vi "DatasheetPrinter.vi"(8 "Temp":i32[](array[numeric]), 9 "Retest":i32[](array[numeric]), 10 "Data_P_F":i8[](array[numeric]), 11 "Data":sgl[](array[numeric])) -> ()   [LabVIEW 2023]
uses:
  Datasheet.ctl
panel:
  in  "Log Name":string
  in  "SN":string
  in  "Tube Type":string
  in  "Operator":string
  in  "Datasheet":T1={"Large FS Tests"=0, "Small FS Tests"=1, "TYPE:"="", "SN:"="", "Retest1"="0", "C"=0.0, "Retest2"="0", "C2"=0.0, "Retest3"="0", "C3"=0.0, "Retest4"="0", "C4"=0.0, "Retest5"="0", "C5"=0.0, "Retest6"="0", "C6"=0.0, "Retest7"="0", "C7"=0.0, "Retest10"="0", "C10"=0.0, "Retest13"="0", "C13"=0.0, "Retest19"="0", "C19"=0.0, "Retest25"="0", "C25"=0.0, "Retest29"="0", "C29"=0.0, "Retest33"="0", "C33"=0.0, "Retest37"="0", "C37"=0.0, "Retest41"="0", "C41"=0.0, "Retest45"="0", "C45"=0.0, "Retest57"="0", "C57"=0.0, "Retest61"="0", "C61"=0.0, "Log Name:"="", "Date"="", "Time"="", "OP:"=""}
  # "Temp"
  # "01"
  # "02"
  # "03"
  # "04"
  # "05"
  # "06"
  # "08"
  # "09"
  # "07"
  # "11"
  # "12"
  # "10"
  # "14"
  # "15"
  # "13"
  # "20"
  # "21"
  # "19"
  # "26"
  # "27"
  # "28"
  # "25"
  # "30"
  # "31"
  # "29"
  # "32"
  # "34"
  # "35"
  # "33"
  # "36"
  # "38"
  # "39"
  # "37"
  # "40"
  # "42"
  # "43"
  # "41"
  # "44"
  # "46"
  # "47"
  # "45"
  # "48"
  # "58"
  # "59"
  # "60"
  # "57"
  # "62"
  # "63"
  # "64"
  # "61"
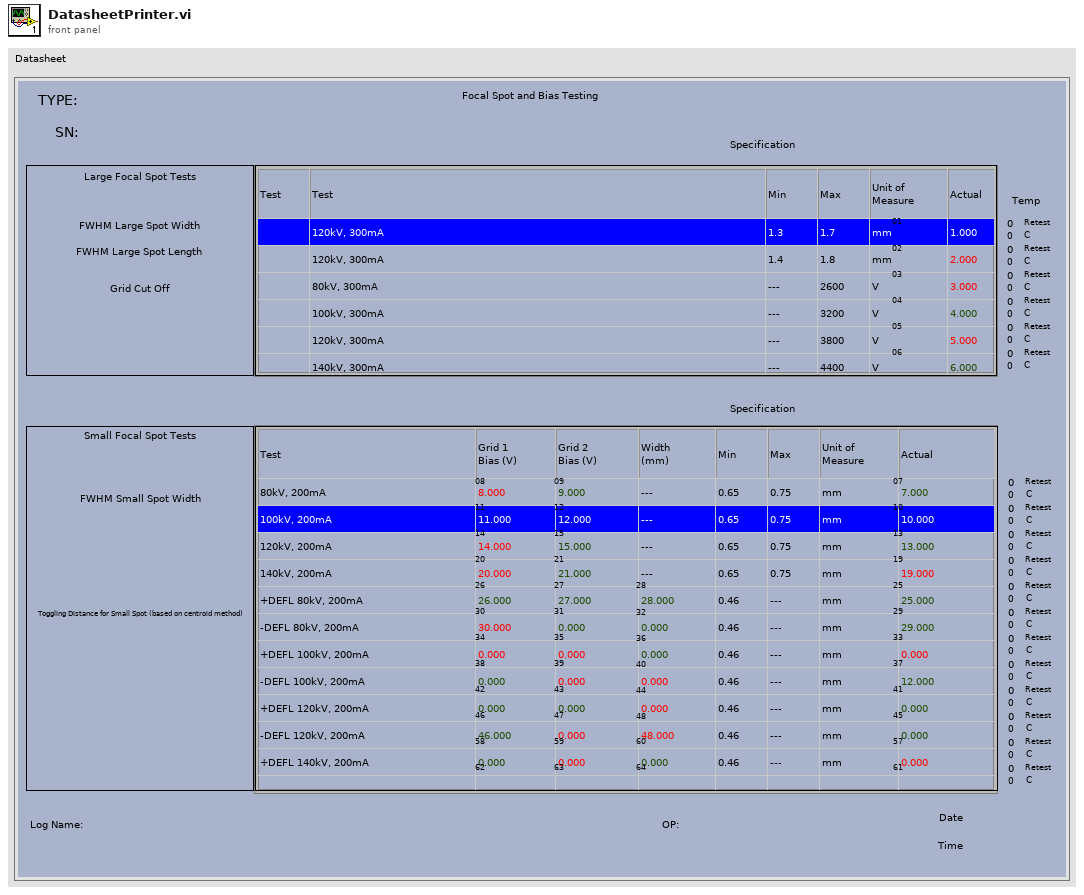
[diagram p1: front panel]
types:
  T1 = typedef "Datasheet.ctl" = cluster{"Large FS Tests":i32, "Small FS Tests":i32, "TYPE:":string, "SN:":string, "Retest1":string, "C":dbl, "Retest2":string, "C2":dbl, "Retest3":string, "C3":dbl, "Retest4":string, "C4":dbl, "Retest5":string, "C5":dbl, "Retest6":string, "C6":dbl, "Retest7":string, "C7":dbl, "Retest10":string, "C10":dbl, "Retest13":string, "C13":dbl, "Retest19":string, "C19":dbl, "Retest25":string, "C25":dbl, "Retest29":string, "C29":dbl, "Retest33":string, "C33":dbl, "Retest37":string, "C37":dbl, "Retest41":string, "C41":dbl, "Retest45":string, "C45":dbl, "Retest57":string, "C57":dbl, "Retest61":string, "C61":dbl, "Log Name:":string, "Date":string, "Time":string, "OP:":string}
  T2 = cluster{"Temp[0]":i32, "Temp[1]":i32, "Temp[2]":i32, "Temp[3]":i32, "Temp[4]":i32, "Temp[5]":i32, "Temp[6]":i32, "Temp[7]":i32, "Temp[8]":i32, "Temp[9]":i32, "Temp[10]":i32, "Temp[11]":i32, "Temp[12]":i32, "Temp[13]":i32, "Temp[14]":i32, "Temp[15]":i32, "Temp[16]":i32, "Temp[17]":i32}
  T3 = cluster{"[0]":string, "[1]":string, "[2]":string, "[3]":string, "[4]":string, "[5]":string, "[6]":string, "[7]":string, "[8]":string, "[9]":string, "[10]":string, "[11]":string, "[12]":string, "[13]":string, "[14]":string, "[15]":string, "[16]":string, "[17]":string}
  T4 = typedef "LVRowAndColumnTypeDef.ctl" = cluster{"Row":i32, "Column":i32}
  T5 = typedef "imagedata.ctl" = cluster{"image type":i32, "image depth":i32, "image":u8[], "mask":u8[], "colors":u32[], "Rectangle":cluster{"left":i16, "top":i16, "right":i16, "bottom":i16}}
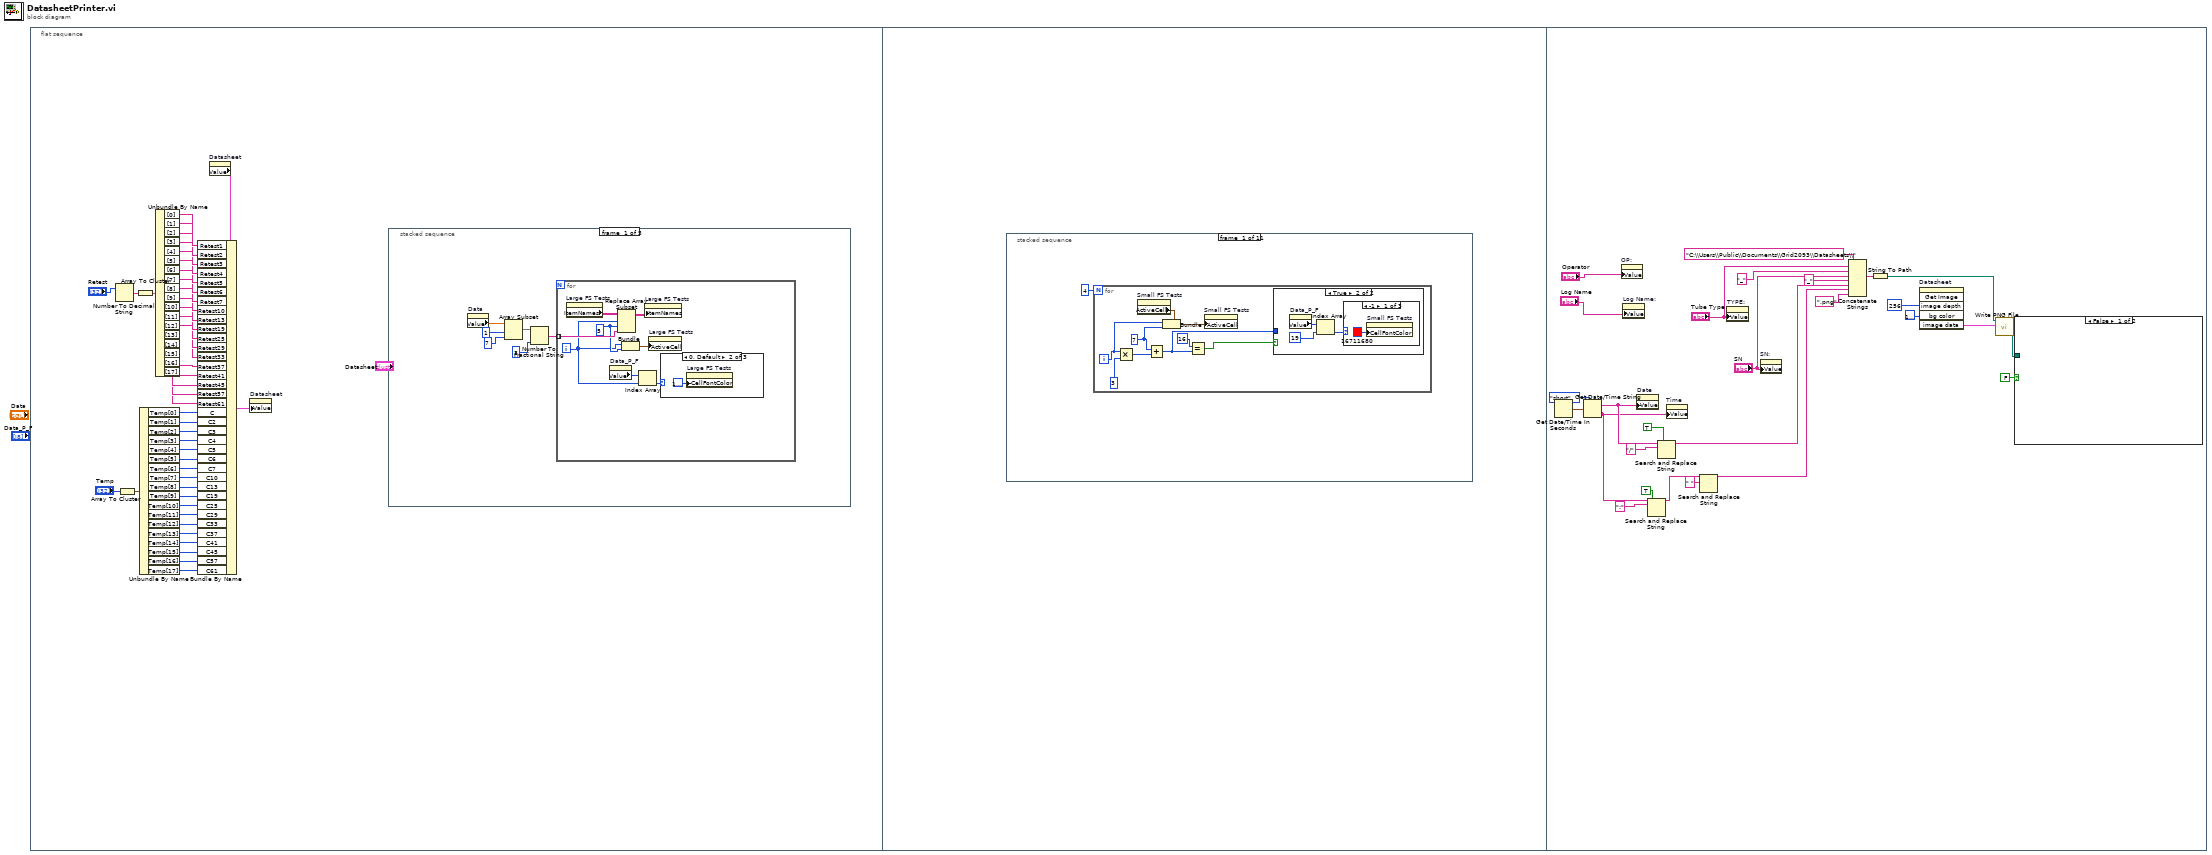
[diagram p0: block diagram]
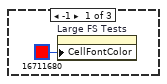
[diagram p2: hidden frame]
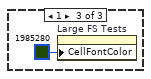
[diagram p3: hidden frame]
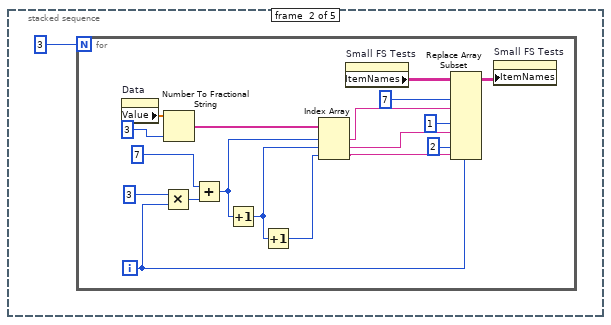
[diagram p4: hidden frame]
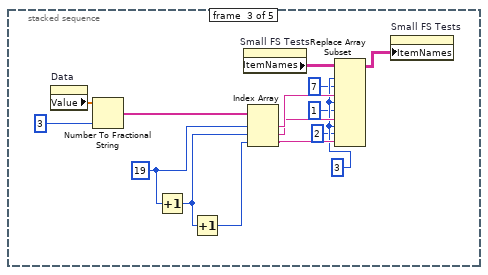
[diagram p5: hidden frame]
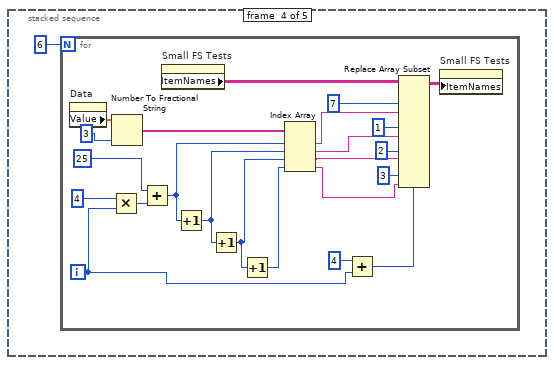
[diagram p6: hidden frame]
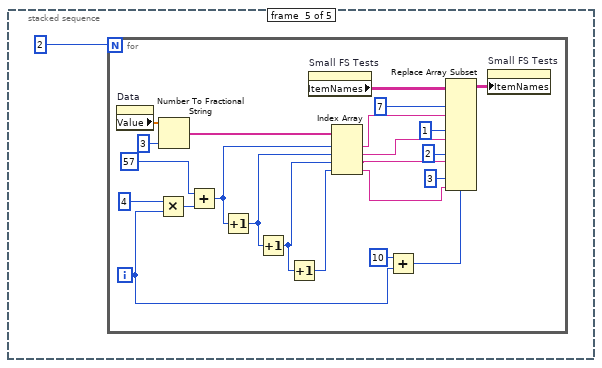
[diagram p7: hidden frame]
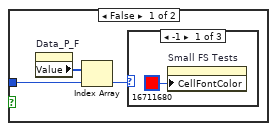
[diagram p8: hidden frame]
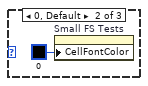
[diagram p9: hidden frame]
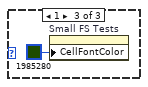
[diagram p10: hidden frame]
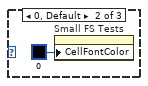
[diagram p11: hidden frame]
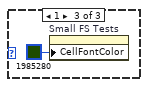
[diagram p12: hidden frame]
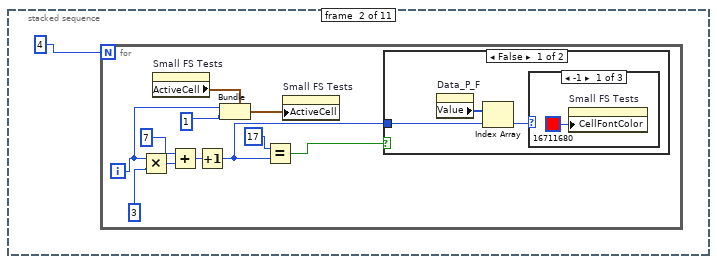
[diagram p13: hidden frame]
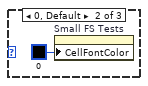
[diagram p14: hidden frame]
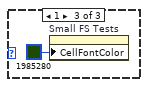
[diagram p15: hidden frame]
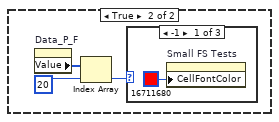
[diagram p16: hidden frame]
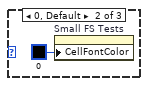
[diagram p17: hidden frame]
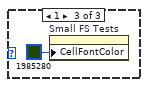
[diagram p18: hidden frame]
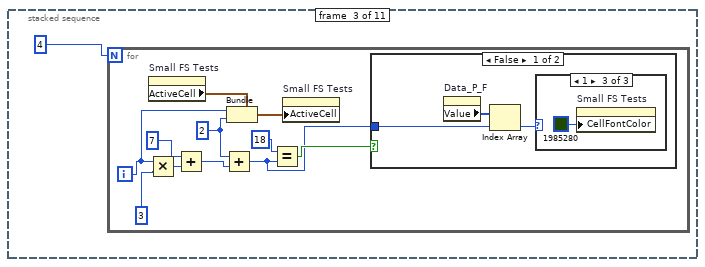
[diagram p19: hidden frame]
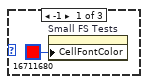
[diagram p20: hidden frame]
diagram:
  n1 = flat-sequence {
    frame #0 {
      n2 = Number To Decimal String(number="Retest") -> (decimal integer string=w40:string[])  [unwired: 1 in]
      n3 = Array To Cluster(array="Temp") -> (cluster=w19:T2)
      n4 = Array To Cluster(array=w40) -> (cluster=w39:T3)
      n5 = Unbundle By Name(w19) -> ("Temp[0]"=w18:i32, "Temp[1]"=w17:i32, "Temp[2]"=w16:i32, "Temp[3]"=w15:i32, "Temp[4]"=w14:i32, "Temp[5]"=w13:i32, "Temp[6]"=w12:i32, "Temp[7]"=w11:i32, "Temp[8]"=w10:i32, "Temp[9]"=w9:i32, "Temp[10]"=w8:i32, "Temp[11]"=w7:i32, "Temp[12]"=w6:i32, "Temp[13]"=w5:i32, "Temp[14]"=w4:i32, "Temp[15]"=w3:i32, "Temp[16]"=w2:i32, "Temp[17]"=w1:i32)
      n6 = Unbundle By Name(w39) -> ("[0]"=w38:string, "[1]"=w37:string, "[2]"=w36:string, "[3]"=w35:string, "[4]"=w34:string, "[5]"=w33:string, "[6]"=w32:string, "[7]"=w31:string, "[8]"=w30:string, "[9]"=w29:string, "[10]"=w28:string, "[11]"=w27:string, "[12]"=w26:string, "[13]"=w25:string, "[14]"=w24:string, "[15]"=w23:string, "[16]"=w22:string, "[17]"=w21:string)
      n7 = property on="Datasheet" class="Clust (strict)"() -> ("Value"=w42:T1)  [unwired: 2 in, 2 out]
      n8 = Bundle By Name(cluster=w42, "Retest1"=w38, "Retest2"=w37, "Retest3"=w36, "Retest4"=w35, "Retest5"=w34, "Retest6"=w33, "Retest7"=w32, "Retest10"=w31, "Retest13"=w30, "Retest19"=w29, "Retest25"=w28, "Retest29"=w27, "Retest33"=w26, "Retest37"=w25, "Retest41"=w24, "Retest45"=w23, "Retest57"=w22, "Retest61"=w21, "C"=w18, "C2"=w17, "C3"=w16, "C4"=w15, "C5"=w14, "C6"=w13, "C7"=w12, "C10"=w11, "C13"=w10, "C19"=w9, "C25"=w8, "C29"=w7, "C33"=w6, "C37"=w5, "C41"=w4, "C45"=w3, "C57"=w2, "C61"=w1) -> (w43:T1)
      n9 = property on="Datasheet" class="Clust (strict)"("Value"=w43) -> ()  [unwired: 2 in, 2 out]
      n10 = stacked-sequence {
        frame #0 {
          n11 = property on="Data" class="Arr (strict)"() -> ("Value"=w47:sgl[])  [unwired: 2 in, 2 out]
          n12 = Array Subset(array=w47, index=1, length=7) -> (w48:sgl[])
          n13 = Number To Fractional String(number=w48, precision (6)=i16 3) -> (F-format string=w49:string[])  [unwired: 2 in]
          n14 = for {
            tunnel: w49 -> [w57] mode=indexing
            i -> [w50]
            w52 = 5 ("index (col)")
            n15 = property on="Large FS Tests" class="MCListbox (strict)"() -> ("ItemNames"=w56:string[][])  [unwired: 2 in, 2 out]
            n16 = property on="Data_P_F" class="Arr (strict)"() -> ("Value"=w54:i8[])  [unwired: 2 in, 2 out]
            n17 = Replace Array Subset(array=w56, new element=w57, index (row)=w50, index (col)=w52) -> (w55:string[][])
            n18 = Bundle(w50, "index (col)"=w52) -> (w51:cluster{i32, "index (col)":i32})  [unwired: 1 in]
            n19 = Index Array(array=w54, index=w50) -> (element=w53:i8)
            n20 = property on="Large FS Tests" class="MCListbox (strict)"("ItemNames"=w55) -> ()  [unwired: 2 in, 2 out]
            n21 = property on="Large FS Tests" class="MCListbox (strict)"("ActiveCell"=w51) -> ()  [unwired: 2 in, 2 out]
            n22 = case shown="0, Default" w53 {
              frame -1 {
                n23 = property on="Large FS Tests" class="MCListbox (strict)"("CellFontColor"=u32 16711680 ("Active Cell:Cell Font:Color")) -> ()  [unwired: 2 in, 2 out]
              }
              frame 0, Default {
                n24 = property on="Large FS Tests" class="MCListbox (strict)"("CellFontColor"=u32 16777222 ("Active Cell:Cell Font:Color")) -> ()  [unwired: 2 in, 2 out]
              }
              frame 1 {
                n25 = property on="Large FS Tests" class="MCListbox (strict)"("CellFontColor"=u32 1985280 ("Active Cell:Cell Font:Color")) -> ()  [unwired: 2 in, 2 out]
              }
            }
          }
        }
        frame #1 {
          n26 = for {
            N: 3 -> [_]
            i -> [w68]
            n27 = property on="Data" class="Arr (strict)"() -> ("Value"=w74:sgl[])  [unwired: 2 in, 2 out]
            n28 = Multiply(x=3, y=w68) -> (x*y=w76:i32)
            n29 = Number To Fractional String(number=w74, precision (6)=i16 3) -> (F-format string=w73:string[])  [unwired: 2 in]
            n30 = Add(x=7, y=w76) -> (x+y=w75:i32)
            n31 = Increment(x=w75) -> (x+1=w67:i32)
            n32 = Increment(x=w67) -> (x+1=w66:i32)
            n33 = Index Array(array=w73, index #1=w75, index #2=w67, index #3=w66) -> (element #1=w72:string, element #2=w65:string, element #3=w64:string)
            n34 = property on="Small FS Tests" class="MCListbox (strict)"() -> ("ItemNames"=w79:string[][])  [unwired: 2 in, 2 out]
            n35 = Replace Array Subset(array=w79, new element #1=w72, index (row) #1=w68, index (col) #1=7 ("index (col)"), new element #2=w65, index (row) #2=w68, index (col) #2=1 ("index (col)"), new element #3=w64, index (row) #3=w68, index (col) #3=2 ("index (col)")) -> (w62:string[][])
            n36 = property on="Small FS Tests" class="MCListbox (strict)"("ItemNames"=w62) -> ()  [unwired: 2 in, 2 out]
          }
        }
        frame #2 {
          w84 = 19 ("x")
          w83 = 3 ("index (row)")
          n37 = property on="Data" class="Arr (strict)"() -> ("Value"=w92:sgl[])  [unwired: 2 in, 2 out]
          n38 = Number To Fractional String(number=w92, precision (6)=i16 3) -> (F-format string=w91:string[])  [unwired: 2 in]
          n39 = Increment(x=w84) -> (x+1=w89:i32)
          n40 = Increment(x=w89) -> (x+1=w88:i32)
          n41 = property on="Small FS Tests" class="MCListbox (strict)"() -> ("ItemNames"=w93:string[][])  [unwired: 2 in, 2 out]
          n42 = Index Array(array=w91, index #1=w84, index #2=w89, index #3=w88) -> (element #1=w90:string, element #2=w87:string, element #3=w86:string)
          n43 = Replace Array Subset(array=w93, new element #1=w90, index (row) #1=w83, index (col) #1=7 ("index (col)"), new element #2=w87, index (row) #2=w83, index (col) #2=1 ("index (col)"), new element #3=w86, index (row) #3=w83, index (col) #3=2 ("index (col)")) -> (w94:string[][])
          n44 = property on="Small FS Tests" class="MCListbox (strict)"("ItemNames"=w94) -> ()  [unwired: 2 in, 2 out]
        }
        frame #3 {
          n45 = for {
            N: 6 -> [_]
            i -> [w100]
            n46 = property on="Data" class="Arr (strict)"() -> ("Value"=w114:sgl[])  [unwired: 2 in, 2 out]
            n47 = Multiply(x=4, y=w100) -> (x*y=w116:i32)
            n48 = Number To Fractional String(number=w114, precision (6)=i16 3) -> (F-format string=w113:string[])  [unwired: 2 in]
            n49 = Add(x=25, y=w116) -> (x+y=w115:i32)
            n50 = property on="Small FS Tests" class="MCListbox (strict)"() -> ("ItemNames"=w96:string[][])  [unwired: 2 in, 2 out]
            n51 = Increment(x=w115) -> (x+1=w108:i32)
            n52 = Increment(x=w108) -> (x+1=w104:i32)
            n53 = Increment(x=w104) -> (x+1=w103:i32)
            n54 = Index Array(array=w113, index #1=w115, index #2=w108, index #3=w104, index #4=w103) -> (element #1=w112:string, element #2=w107:string, element #3=w106:string, element #4=w102:string)
            n55 = Add(x=4, y=w100) -> (x+y=w99:i32)
            n56 = Replace Array Subset(array=w96, new element #1=w112, index (row) #1=w99, index (col) #1=7 ("index (col)"), new element #2=w107, index (row) #2=w99, index (col) #2=1 ("index (col)"), new element #3=w106, index (row) #3=w99, index (col) #3=2 ("index (col)"), new element #4=w102, index (row) #4=w99, index (col) #4=3 ("index (col)")) -> (w97:string[][])
            n57 = property on="Small FS Tests" class="MCListbox (strict)"("ItemNames"=w97) -> ()  [unwired: 2 in, 2 out]
          }
        }
        frame #4 {
          n58 = for {
            N: 2 -> [_]
            i -> [w123]
            n59 = property on="Data" class="Arr (strict)"() -> ("Value"=w138:sgl[])  [unwired: 2 in, 2 out]
            n60 = Multiply(x=4, y=w123) -> (x*y=w140:i32)
            n61 = Number To Fractional String(number=w138, precision (6)=i16 3) -> (F-format string=w137:string[])  [unwired: 2 in]
            n62 = Add(x=57, y=w140) -> (x+y=w139:i32)
            n63 = Increment(x=w139) -> (x+1=w131:i32)
            n64 = Increment(x=w131) -> (x+1=w127:i32)
            n65 = Increment(x=w127) -> (x+1=w126:i32)
            n66 = property on="Small FS Tests" class="MCListbox (strict)"() -> ("ItemNames"=w120:string[][])  [unwired: 2 in, 2 out]
            n67 = Index Array(array=w137, index #1=w139, index #2=w131, index #3=w127, index #4=w126) -> (element #1=w136:string, element #2=w130:string, element #3=w129:string, element #4=w125:string)
            n68 = Add(x=10, y=w123) -> (x+y=w122:i32)
            n69 = Replace Array Subset(array=w120, new element #1=w136, index (row) #1=w122, index (col) #1=7 ("index (col)"), new element #2=w130, index (row) #2=w122, index (col) #2=1 ("index (col)"), new element #3=w129, index (row) #3=w122, index (col) #3=2 ("index (col)"), new element #4=w125, index (row) #4=w122, index (col) #4=3 ("index (col)")) -> (w132:string[][])
            n70 = property on="Small FS Tests" class="MCListbox (strict)"("ItemNames"=w132) -> ()  [unwired: 2 in, 2 out]
          }
        }
      }
    }
    frame #1 {
      n71 = stacked-sequence {
        frame #0 {
          n72 = for {
            N: 4 -> [_]
            i -> [w145]
            w148 = 7 ("x")
            n73 = Multiply(x=w145, y=3 ("x")) -> (x*y=w152:i32)
            n74 = property on="Small FS Tests" class="MCListbox (strict)"() -> ("ActiveCell"=w144:T4)  [unwired: 2 in, 2 out]
            n75 = Add(x=w148, y=w152) -> (x+y=w146:i32)
            n76 = Bundle(cluster=w144, "Row"=w145, "Column"=w148) -> (w147:T4)
            n77 = Equal?(x=16, y=w146) -> (x = y?=w150:bool)
            n78 = property on="Small FS Tests" class="MCListbox (strict)"("ActiveCell"=w147) -> ()  [unwired: 2 in, 2 out]
            n79 = case shown="True" w150 {
              tunnel: w146 -> [w154 _]
              frame False {
                n80 = property on="Data_P_F" class="Arr (strict)"() -> ("Value"=w155:i8[])  [unwired: 2 in, 2 out]
                n81 = Index Array(array=w155, index=w154) -> (element=w153:i8)
                n82 = case shown="-1" w153 {
                  frame -1 {
                    n83 = property on="Small FS Tests" class="MCListbox (strict)"("CellFontColor"=u32 16711680 ("Active Cell:Cell Font:Color")) -> ()  [unwired: 2 in, 2 out]
                  }
                  frame 0, Default {
                    n84 = property on="Small FS Tests" class="MCListbox (strict)"("CellFontColor"=u32 0 ("Active Cell:Cell Font:Color")) -> ()  [unwired: 2 in, 2 out]
                  }
                  frame 1 {
                    n85 = property on="Small FS Tests" class="MCListbox (strict)"("CellFontColor"=u32 1985280 ("Active Cell:Cell Font:Color")) -> ()  [unwired: 2 in, 2 out]
                  }
                }
              }
              frame True {
                n86 = property on="Data_P_F" class="Arr (strict)"() -> ("Value"=w161:i8[])  [unwired: 2 in, 2 out]
                n87 = Index Array(array=w161, index=19) -> (element=w160:i8)
                n88 = case shown="-1" w160 {
                  frame -1 {
                    n89 = property on="Small FS Tests" class="MCListbox (strict)"("CellFontColor"=u32 16711680 ("Active Cell:Cell Font:Color")) -> ()  [unwired: 2 in, 2 out]
                  }
                  frame 0, Default {
                    n90 = property on="Small FS Tests" class="MCListbox (strict)"("CellFontColor"=u32 0 ("Active Cell:Cell Font:Color")) -> ()  [unwired: 2 in, 2 out]
                  }
                  frame 1 {
                    n91 = property on="Small FS Tests" class="MCListbox (strict)"("CellFontColor"=u32 1985280 ("Active Cell:Cell Font:Color")) -> ()  [unwired: 2 in, 2 out]
                  }
                }
              }
            }
          }
        }
        frame #1 {
          n92 = for {
            N: 4 -> [_]
            i -> [w167]
            n93 = Multiply(x=w167, y=3 ("x")) -> (x*y=w176:i32)
            n94 = property on="Small FS Tests" class="MCListbox (strict)"() -> ("ActiveCell"=w166:T4)  [unwired: 2 in, 2 out]
            n95 = Add(x=7, y=w176) -> (x+y=w170:i32)
            n96 = Increment(x=w170) -> (x+1=w169:i32)
            n97 = Bundle(cluster=w166, "Row"=w167, "Column"=1 ("x")) -> (w171:T4)
            n98 = Equal?(x=17, y=w169) -> (x = y?=w174:bool)
            n99 = property on="Small FS Tests" class="MCListbox (strict)"("ActiveCell"=w171) -> ()  [unwired: 2 in, 2 out]
            n100 = case shown="False" w174 {
              tunnel: w169 -> [w178 _]
              frame False {
                n101 = property on="Data_P_F" class="Arr (strict)"() -> ("Value"=w179:i8[])  [unwired: 2 in, 2 out]
                n102 = Index Array(array=w179, index=w178) -> (element=w177:i8)
                n103 = case shown="-1" w177 {
                  frame -1 {
                    n104 = property on="Small FS Tests" class="MCListbox (strict)"("CellFontColor"=u32 16711680 ("Active Cell:Cell Font:Color")) -> ()  [unwired: 2 in, 2 out]
                  }
                  frame 0, Default {
                    n105 = property on="Small FS Tests" class="MCListbox (strict)"("CellFontColor"=u32 0 ("Active Cell:Cell Font:Color")) -> ()  [unwired: 2 in, 2 out]
                  }
                  frame 1 {
                    n106 = property on="Small FS Tests" class="MCListbox (strict)"("CellFontColor"=u32 1985280 ("Active Cell:Cell Font:Color")) -> ()  [unwired: 2 in, 2 out]
                  }
                }
              }
              frame True {
                n107 = property on="Data_P_F" class="Arr (strict)"() -> ("Value"=w185:i8[])  [unwired: 2 in, 2 out]
                n108 = Index Array(array=w185, index=20) -> (element=w184:i8)
                n109 = case shown="-1" w184 {
                  frame -1 {
                    n110 = property on="Small FS Tests" class="MCListbox (strict)"("CellFontColor"=u32 16711680 ("Active Cell:Cell Font:Color")) -> ()  [unwired: 2 in, 2 out]
                  }
                  frame 0, Default {
                    n111 = property on="Small FS Tests" class="MCListbox (strict)"("CellFontColor"=u32 0 ("Active Cell:Cell Font:Color")) -> ()  [unwired: 2 in, 2 out]
                  }
                  frame 1 {
                    n112 = property on="Small FS Tests" class="MCListbox (strict)"("CellFontColor"=u32 1985280 ("Active Cell:Cell Font:Color")) -> ()  [unwired: 2 in, 2 out]
                  }
                }
              }
            }
          }
        }
        frame #2 {
          n113 = for {
            N: 4 -> [_]
            i -> [w191]
            w192 = 2 ("x")
            n114 = Multiply(x=w191, y=3 ("x")) -> (x*y=w200:i32)
            n115 = property on="Small FS Tests" class="MCListbox (strict)"() -> ("ActiveCell"=w190:T4)  [unwired: 2 in, 2 out]
            n116 = Add(x=7, y=w200) -> (x+y=w193:i32)
            n117 = Add(x=w192, y=w193) -> (x+y=w194:i32)
            n118 = Bundle(cluster=w190, "Row"=w191, "Column"=w192) -> (w195:T4)
            n119 = Equal?(x=18, y=w194) -> (x = y?=w198:bool)
            n120 = property on="Small FS Tests" class="MCListbox (strict)"("ActiveCell"=w195) -> ()  [unwired: 2 in, 2 out]
            n121 = case shown="False" w198 {
              tunnel: w194 -> [w202 _]
              frame False {
                n122 = property on="Data_P_F" class="Arr (strict)"() -> ("Value"=w203:i8[])  [unwired: 2 in, 2 out]
                n123 = Index Array(array=w203, index=w202) -> (element=w201:i8)
                n124 = case shown="1" w201 {
                  frame -1 {
                    n125 = property on="Small FS Tests" class="MCListbox (strict)"("CellFontColor"=u32 16711680 ("Active Cell:Cell Font:Color")) -> ()  [unwired: 2 in, 2 out]
                  }
                  frame 0, Default {
                    n126 = property on="Small FS Tests" class="MCListbox (strict)"("CellFontColor"=u32 0 ("Active Cell:Cell Font:Color")) -> ()  [unwired: 2 in, 2 out]
                  }
                  frame 1 {
                    n127 = property on="Small FS Tests" class="MCListbox (strict)"("CellFontColor"=u32 1985280 ("Active Cell:Cell Font:Color")) -> ()  [unwired: 2 in, 2 out]
                  }
                }
              }
              frame True {
                n128 = property on="Data_P_F" class="Arr (strict)"() -> ("Value"=w209:i8[])  [unwired: 2 in, 2 out]
                n129 = Index Array(array=w209, index=21) -> (element=w208:i8)
                n130 = case shown="1" w208 {
                  frame -1 {
                    n131 = property on="Small FS Tests" class="MCListbox (strict)"("CellFontColor"=u32 16711680 ("Active Cell:Cell Font:Color")) -> ()  [unwired: 2 in, 2 out]
                  }
                  frame 0, Default {
                    n132 = property on="Small FS Tests" class="MCListbox (strict)"("CellFontColor"=u32 0 ("Active Cell:Cell Font:Color")) -> ()  [unwired: 2 in, 2 out]
                  }
                  frame 1 {
                    n133 = property on="Small FS Tests" class="MCListbox (strict)"("CellFontColor"=u32 1985280 ("Active Cell:Cell Font:Color")) -> ()  [unwired: 2 in, 2 out]
                  }
                }
              }
            }
          }
        }
        frame #3 {
          n134 = for {
            N: 6 -> [_]
            i -> [w216]
            n135 = Multiply(x=w216, y=4 ("x")) -> (x*y=w225:i32)
            n136 = Add(x=4, y=w216) -> (x+y=w217:i32)
            n137 = property on="Small FS Tests" class="MCListbox (strict)"() -> ("ActiveCell"=w214:T4)  [unwired: 2 in, 2 out]
            n138 = Add(x=25, y=w225) -> (x+y=w222:i32)
            n139 = Bundle(cluster=w214, "Row"=w217, "Column"=7) -> (w219:T4)
            n140 = property on="Small FS Tests" class="MCListbox (strict)"("ActiveCell"=w219) -> ()  [unwired: 2 in, 2 out]
            n141 = property on="Data_P_F" class="Arr (strict)"() -> ("Value"=w221:i8[])  [unwired: 2 in, 2 out]
            n142 = Index Array(array=w221, index=w222) -> (element=w220:i8)
            n143 = case shown="1" w220 {
              frame -1 {
                n144 = property on="Small FS Tests" class="MCListbox (strict)"("CellFontColor"=u32 16711680 ("Active Cell:Cell Font:Color")) -> ()  [unwired: 2 in, 2 out]
              }
              frame 0, Default {
                n145 = property on="Small FS Tests" class="MCListbox (strict)"("CellFontColor"=u32 0 ("Active Cell:Cell Font:Color")) -> ()  [unwired: 2 in, 2 out]
              }
              frame 1 {
                n146 = property on="Small FS Tests" class="MCListbox (strict)"("CellFontColor"=u32 1985280 ("Active Cell:Cell Font:Color")) -> ()  [unwired: 2 in, 2 out]
              }
            }
          }
        }
        frame #4 {
          n147 = for {
            N: 6 -> [_]
            i -> [w232]
            n148 = Multiply(x=w232, y=4 ("x")) -> (x*y=w242:i32)
            n149 = Add(x=4, y=w232) -> (x+y=w233:i32)
            n150 = property on="Small FS Tests" class="MCListbox (strict)"() -> ("ActiveCell"=w230:T4)  [unwired: 2 in, 2 out]
            n151 = Add(x=25, y=w242) -> (x+y=w239:i32)
            n152 = Bundle(cluster=w230, "Row"=w233, "Column"=1) -> (w236:T4)
            n153 = Increment(x=w239) -> (x+1=w234:i32)
            n154 = property on="Small FS Tests" class="MCListbox (strict)"("ActiveCell"=w236) -> ()  [unwired: 2 in, 2 out]
            n155 = property on="Data_P_F" class="Arr (strict)"() -> ("Value"=w238:i8[])  [unwired: 2 in, 2 out]
            n156 = Index Array(array=w238, index=w234) -> (element=w237:i8)
            n157 = case shown="1" w237 {
              frame -1 {
                n158 = property on="Small FS Tests" class="MCListbox (strict)"("CellFontColor"=u32 16711680 ("Active Cell:Cell Font:Color")) -> ()  [unwired: 2 in, 2 out]
              }
              frame 0, Default {
                n159 = property on="Small FS Tests" class="MCListbox (strict)"("CellFontColor"=u32 0 ("Active Cell:Cell Font:Color")) -> ()  [unwired: 2 in, 2 out]
              }
              frame 1 {
                n160 = property on="Small FS Tests" class="MCListbox (strict)"("CellFontColor"=u32 1985280 ("Active Cell:Cell Font:Color")) -> ()  [unwired: 2 in, 2 out]
              }
            }
          }
        }
        frame #5 {
          n161 = for {
            N: 6 -> [_]
            i -> [w249]
            n162 = Multiply(x=w249, y=4 ("x")) -> (x*y=w260:i32)
            n163 = Add(x=4, y=w249) -> (x+y=w250:i32)
            n164 = property on="Small FS Tests" class="MCListbox (strict)"() -> ("ActiveCell"=w247:T4)  [unwired: 2 in, 2 out]
            n165 = Add(x=25, y=w260) -> (x+y=w257:i32)
            n166 = Bundle(cluster=w247, "Row"=w250, "Column"=2) -> (w254:T4)
            n167 = property on="Small FS Tests" class="MCListbox (strict)"("ActiveCell"=w254) -> ()  [unwired: 2 in, 2 out]
            n168 = Add(x=w257, y=2) -> (x+y=w252:i32)
            n169 = property on="Data_P_F" class="Arr (strict)"() -> ("Value"=w256:i8[])  [unwired: 2 in, 2 out]
            n170 = Index Array(array=w256, index=w252) -> (element=w255:i8)
            n171 = case shown="-1" w255 {
              frame -1 {
                n172 = property on="Small FS Tests" class="MCListbox (strict)"("CellFontColor"=u32 16711680 ("Active Cell:Cell Font:Color")) -> ()  [unwired: 2 in, 2 out]
              }
              frame 0, Default {
                n173 = property on="Small FS Tests" class="MCListbox (strict)"("CellFontColor"=u32 0 ("Active Cell:Cell Font:Color")) -> ()  [unwired: 2 in, 2 out]
              }
              frame 1 {
                n174 = property on="Small FS Tests" class="MCListbox (strict)"("CellFontColor"=u32 1985280 ("Active Cell:Cell Font:Color")) -> ()  [unwired: 2 in, 2 out]
              }
            }
          }
        }
        frame #6 {
          n175 = for {
            N: 6 -> [_]
            i -> [w267]
            n176 = Multiply(x=w267, y=4 ("x")) -> (x*y=w278:i32)
            n177 = Add(x=4, y=w267) -> (x+y=w268:i32)
            n178 = property on="Small FS Tests" class="MCListbox (strict)"() -> ("ActiveCell"=w265:T4)  [unwired: 2 in, 2 out]
            n179 = Add(x=25, y=w278) -> (x+y=w275:i32)
            n180 = Bundle(cluster=w265, "Row"=w268, "Column"=3) -> (w272:T4)
            n181 = property on="Small FS Tests" class="MCListbox (strict)"("ActiveCell"=w272) -> ()  [unwired: 2 in, 2 out]
            n182 = Add(x=w275, y=3) -> (x+y=w270:i32)
            n183 = property on="Data_P_F" class="Arr (strict)"() -> ("Value"=w274:i8[])  [unwired: 2 in, 2 out]
            n184 = Index Array(array=w274, index=w270) -> (element=w273:i8)
            n185 = case shown="-1" w273 {
              frame -1 {
                n186 = property on="Small FS Tests" class="MCListbox (strict)"("CellFontColor"=u32 16711680 ("Active Cell:Cell Font:Color")) -> ()  [unwired: 2 in, 2 out]
              }
              frame 0, Default {
                n187 = property on="Small FS Tests" class="MCListbox (strict)"("CellFontColor"=u32 0 ("Active Cell:Cell Font:Color")) -> ()  [unwired: 2 in, 2 out]
              }
              frame 1 {
                n188 = property on="Small FS Tests" class="MCListbox (strict)"("CellFontColor"=u32 1985280 ("Active Cell:Cell Font:Color")) -> ()  [unwired: 2 in, 2 out]
              }
            }
          }
        }
        frame #7 {
          n189 = for {
            N: 2 -> [_]
            i -> [w285]
            n190 = Multiply(x=w285, y=4 ("x")) -> (x*y=w294:i32)
            n191 = Add(x=10, y=w285) -> (x+y=w286:i32)
            n192 = property on="Small FS Tests" class="MCListbox (strict)"() -> ("ActiveCell"=w283:T4)  [unwired: 2 in, 2 out]
            n193 = Add(x=57, y=w294) -> (x+y=w291:i32)
            n194 = Bundle(cluster=w283, "Row"=w286, "Column"=7) -> (w288:T4)
            n195 = property on="Small FS Tests" class="MCListbox (strict)"("ActiveCell"=w288) -> ()  [unwired: 2 in, 2 out]
            n196 = property on="Data_P_F" class="Arr (strict)"() -> ("Value"=w290:i8[])  [unwired: 2 in, 2 out]
            n197 = Index Array(array=w290, index=w291) -> (element=w289:i8)
            n198 = case shown="1" w289 {
              frame -1 {
                n199 = property on="Small FS Tests" class="MCListbox (strict)"("CellFontColor"=u32 16711680 ("Active Cell:Cell Font:Color")) -> ()  [unwired: 2 in, 2 out]
              }
              frame 0, Default {
                n200 = property on="Small FS Tests" class="MCListbox (strict)"("CellFontColor"=u32 0 ("Active Cell:Cell Font:Color")) -> ()  [unwired: 2 in, 2 out]
              }
              frame 1 {
                n201 = property on="Small FS Tests" class="MCListbox (strict)"("CellFontColor"=u32 1985280 ("Active Cell:Cell Font:Color")) -> ()  [unwired: 2 in, 2 out]
              }
            }
          }
        }
        frame #8 {
          n202 = for {
            N: 2 -> [_]
            i -> [w301]
            n203 = Multiply(x=w301, y=4 ("x")) -> (x*y=w311:i32)
            n204 = Add(x=10, y=w301) -> (x+y=w302:i32)
            n205 = property on="Small FS Tests" class="MCListbox (strict)"() -> ("ActiveCell"=w299:T4)  [unwired: 2 in, 2 out]
            n206 = Add(x=57, y=w311) -> (x+y=w308:i32)
            n207 = Bundle(cluster=w299, "Row"=w302, "Column"=1) -> (w305:T4)
            n208 = Increment(x=w308) -> (x+1=w303:i32)
            n209 = property on="Small FS Tests" class="MCListbox (strict)"("ActiveCell"=w305) -> ()  [unwired: 2 in, 2 out]
            n210 = property on="Data_P_F" class="Arr (strict)"() -> ("Value"=w307:i8[])  [unwired: 2 in, 2 out]
            n211 = Index Array(array=w307, index=w303) -> (element=w306:i8)
            n212 = case shown="1" w306 {
              frame -1 {
                n213 = property on="Small FS Tests" class="MCListbox (strict)"("CellFontColor"=u32 16711680 ("Active Cell:Cell Font:Color")) -> ()  [unwired: 2 in, 2 out]
              }
              frame 0, Default {
                n214 = property on="Small FS Tests" class="MCListbox (strict)"("CellFontColor"=u32 0 ("Active Cell:Cell Font:Color")) -> ()  [unwired: 2 in, 2 out]
              }
              frame 1 {
                n215 = property on="Small FS Tests" class="MCListbox (strict)"("CellFontColor"=u32 1985280 ("Active Cell:Cell Font:Color")) -> ()  [unwired: 2 in, 2 out]
              }
            }
          }
        }
        frame #9 {
          n216 = for {
            N: 2 -> [_]
            i -> [w318]
            n217 = Multiply(x=w318, y=4 ("x")) -> (x*y=w329:i32)
            n218 = Add(x=10, y=w318) -> (x+y=w319:i32)
            n219 = property on="Small FS Tests" class="MCListbox (strict)"() -> ("ActiveCell"=w316:T4)  [unwired: 2 in, 2 out]
            n220 = Add(x=57, y=w329) -> (x+y=w326:i32)
            n221 = Bundle(cluster=w316, "Row"=w319, "Column"=2) -> (w323:T4)
            n222 = property on="Small FS Tests" class="MCListbox (strict)"("ActiveCell"=w323) -> ()  [unwired: 2 in, 2 out]
            n223 = Add(x=w326, y=2) -> (x+y=w321:i32)
            n224 = property on="Data_P_F" class="Arr (strict)"() -> ("Value"=w325:i8[])  [unwired: 2 in, 2 out]
            n225 = Index Array(array=w325, index=w321) -> (element=w324:i8)
            n226 = case shown="-1" w324 {
              frame -1 {
                n227 = property on="Small FS Tests" class="MCListbox (strict)"("CellFontColor"=u32 16711680 ("Active Cell:Cell Font:Color")) -> ()  [unwired: 2 in, 2 out]
              }
              frame 0, Default {
                n228 = property on="Small FS Tests" class="MCListbox (strict)"("CellFontColor"=u32 0 ("Active Cell:Cell Font:Color")) -> ()  [unwired: 2 in, 2 out]
              }
              frame 1 {
                n229 = property on="Small FS Tests" class="MCListbox (strict)"("CellFontColor"=u32 1985280 ("Active Cell:Cell Font:Color")) -> ()  [unwired: 2 in, 2 out]
              }
            }
          }
        }
        frame #10 {
          n230 = for {
            N: 2 -> [_]
            i -> [w336]
            n231 = Multiply(x=w336, y=4 ("x")) -> (x*y=w347:i32)
            n232 = Add(x=10, y=w336) -> (x+y=w337:i32)
            n233 = property on="Small FS Tests" class="MCListbox (strict)"() -> ("ActiveCell"=w334:T4)  [unwired: 2 in, 2 out]
            n234 = Add(x=57, y=w347) -> (x+y=w344:i32)
            n235 = Bundle(cluster=w334, "Row"=w337, "Column"=3) -> (w341:T4)
            n236 = property on="Small FS Tests" class="MCListbox (strict)"("ActiveCell"=w341) -> ()  [unwired: 2 in, 2 out]
            n237 = Add(x=w344, y=3) -> (x+y=w339:i32)
            n238 = property on="Data_P_F" class="Arr (strict)"() -> ("Value"=w343:i8[])  [unwired: 2 in, 2 out]
            n239 = Index Array(array=w343, index=w339) -> (element=w342:i8)
            n240 = case shown="-1" w342 {
              frame -1 {
                n241 = property on="Small FS Tests" class="MCListbox (strict)"("CellFontColor"=u32 16711680 ("Active Cell:Cell Font:Color")) -> ()  [unwired: 2 in, 2 out]
              }
              frame 0, Default {
                n242 = property on="Small FS Tests" class="MCListbox (strict)"("CellFontColor"=u32 0 ("Active Cell:Cell Font:Color")) -> ()  [unwired: 2 in, 2 out]
              }
              frame 1 {
                n243 = property on="Small FS Tests" class="MCListbox (strict)"("CellFontColor"=u32 1985280 ("Active Cell:Cell Font:Color")) -> ()  [unwired: 2 in, 2 out]
              }
            }
          }
        }
      }
    }
    frame #2 {
      n244 = Get Date/Time In Seconds() -> (seconds since 1Jan1904=w364:timestamp)
      n245 = Get Date/Time String(date format (0)=enum16{"short", "long", "abbreviated"}."short", seconds (now)=w364) -> (date string=w374:string, time string=w373:string)  [unwired: 1 in]
      n246 = property on="OP:" class="Str"("Value"="Operator") -> ()  [unwired: 2 in, 2 out]
      n247 = property on="Log Name:" class="Str"("Value"="Log Name") -> ()  [unwired: 2 in, 2 out]
      n248 = property on="Date" class="Str"("Value"=w374) -> ()  [unwired: 2 in, 2 out]
      n249 = Search and Replace String(replace all?=TRUE ("replace all? (F)"), input string=w373, search string=":") -> (result string=w376:string)  [unwired: 5 in, 3 out]
      n250 = Search and Replace String(replace all?=TRUE ("replace all? (F)"), input string=w374, search string="/") -> (result string=w375:string)  [unwired: 5 in, 3 out]
      n251 = property on="Time" class="Str"("Value"=w373) -> ()  [unwired: 2 in, 2 out]
      n252 = Search and Replace String(input string=w376, search string=" ") -> (result string=w372:string)  [unwired: 6 in, 3 out]
      n253 = property on="TYPE:" class="Str"("Value"="Tube Type") -> ()  [unwired: 2 in, 2 out]
      n254 = property on="SN:" class="Str"("Value"="SN") -> ()  [unwired: 2 in, 2 out]
      n255 = Concatenate Strings("C:\\Users\\Public\\Documents\\Grid2093\\Datasheets\\" ("string"), "Tube Type", "_" ("string"), "SN", "_" ("string"), w375, w372, ".png" ("string")) -> (w370:string)
      n256 = String To Path(string=w370) -> (path=w371:path)
      n257 = invoke on="Datasheet" class="Clust (strict)" method="Get Image"("image depth"=256 ("Image Depth"), "bg color"=u32 16777216 ("Background Color")) -> ("image data"=w367:T5)  [unwired: 4 in, 5 out]
      n258 = call <vilib>:"Write PNG File.vi"("image data"=w367, "path to PNG file"=w371) -> ("path"=w377:path)  [unwired: 8 in, 1 out]
      n259 = case shown="False" FALSE {
        tunnel: w377 -> [_ w378]
        frame False {
        }
        frame True {
          n260 = Path To String(path=w378) -> (string=w380:string)
          n261 = Concatenate Strings("MSPaint /P \"" ("string"), w380, "\"" ("string")) -> (w382:string)
          n262 = call <vilib>:"System Exec.vi"("command line"=w382) -> ()  [unwired: 7 in, 4 out]
        }
      }
    }
  }
